vi "Get Child Tags.vi"(8 "error in (no error)":errorcluster, 10 "parent tag":string, 11 "tree in":refnum<vi>) -> (0 "error out":errorcluster, 2 "child tags":string[](array[string]), 3 "tree out":refnum<vi>)   [LabVIEW 2017]
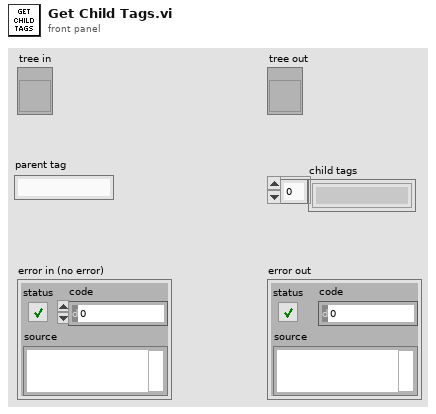
[diagram p1: front panel]
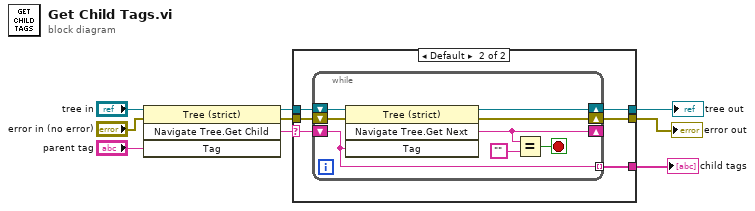
[diagram p0: block diagram]
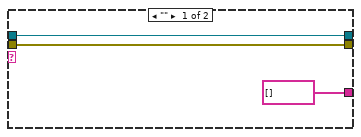
[diagram p2: hidden frame]
diagram:
  n1 = invoke class="Tree (strict)" method="Navigate Tree.Get Child"(reference="tree in", error in="error in (no error)", "Tag"="parent tag") -> (reference out=w6:refnum<vi>, error out=w5:errorcluster, "Navigate Tree:Get Child"=w4:string)  [unwired: 1 in, 1 out]
  n2 = case shown="Default" w4 {
    selector: w4 -> [_ w16]
    tunnel: w6 -> [w11 w18]
    tunnel: w5 -> [w10 w17]
    tunnel: [w10 w15] -> w3
    tunnel: [w11 w14] -> w2
    tunnel: [string[] [] w13] -> w1
    frame "" {
    }
    frame Default {
      n3 = while {
        shift-right: [w24] -> _
        shift-left: w16 -> [w21]
        shift-right: [w20] -> w14
        shift-left: w18 -> [w26]
        shift-right: [w19] -> w15
        shift-left: w17 -> [w25]
        tunnel: [w21] -> w13 mode=indexing
        stop <- w22 stop-if-true
        n4 = invoke class="Tree (strict)" method="Navigate Tree.Get Next"(reference=w26, error in=w25, "Tag"=w21) -> (reference out=w20:refnum<vi>, error out=w19:errorcluster, "Navigate Tree:Get Next Item"=w24:string)  [unwired: 1 in, 1 out]
        n5 = Equal?(x=w24, y="") -> (x = y?=w22:bool)
      }
    }
  }
  "tree out" <- w2
  "error out" <- w3
  "child tags" <- w1
